vi "Get Plot Name Notifier Ref.vi"(8 "error in (no error)":errorcluster) -> (0 "error out":errorcluster, 3 "Plot Names Notifier Ref":refnum<notifier>)   [LabVIEW 2017, in "3D Plot.lvclass"]
uses:
  <vilib>/Math Plots/3D Math Plots/3D Plot/3D Plot/3D Plot.lvclass
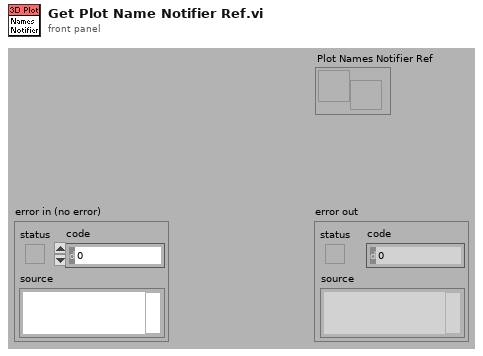
[diagram p1: front panel]
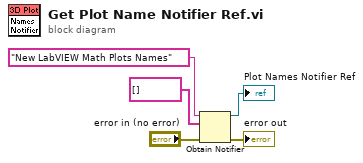
[diagram p0: block diagram]
diagram:
  n1 = Obtain Notifier(name (unnamed)="New LabVIEW Math Plots Names", notification data type=string[] [] ("Appearance Property.Backup Data.Plot Name"), error in (no error)="error in (no error)") -> (notifier out=→"Plot Names Notifier Ref":refnum<notifier>, error out=→"error out":errorcluster)  [unwired: 1 in, 1 out]
